vi "DutLug.vi"() -> (3 "histogram 2":T2(graph))   [LabVIEW 2019]
uses:
  <vilib>/Analysis/NI_AALBase.lvlib
panel:
  out "Cumulative count":cluster{"data sorted":dbl[], i32[]}(graph)
  out "sorted data":dbl[](graph)
  out "linear data out":dbl[](graph)
  out "Dynamic histogram out":T1(graph)
  out "histogram 1":T2(graph)
  in  "intervals":i32=200
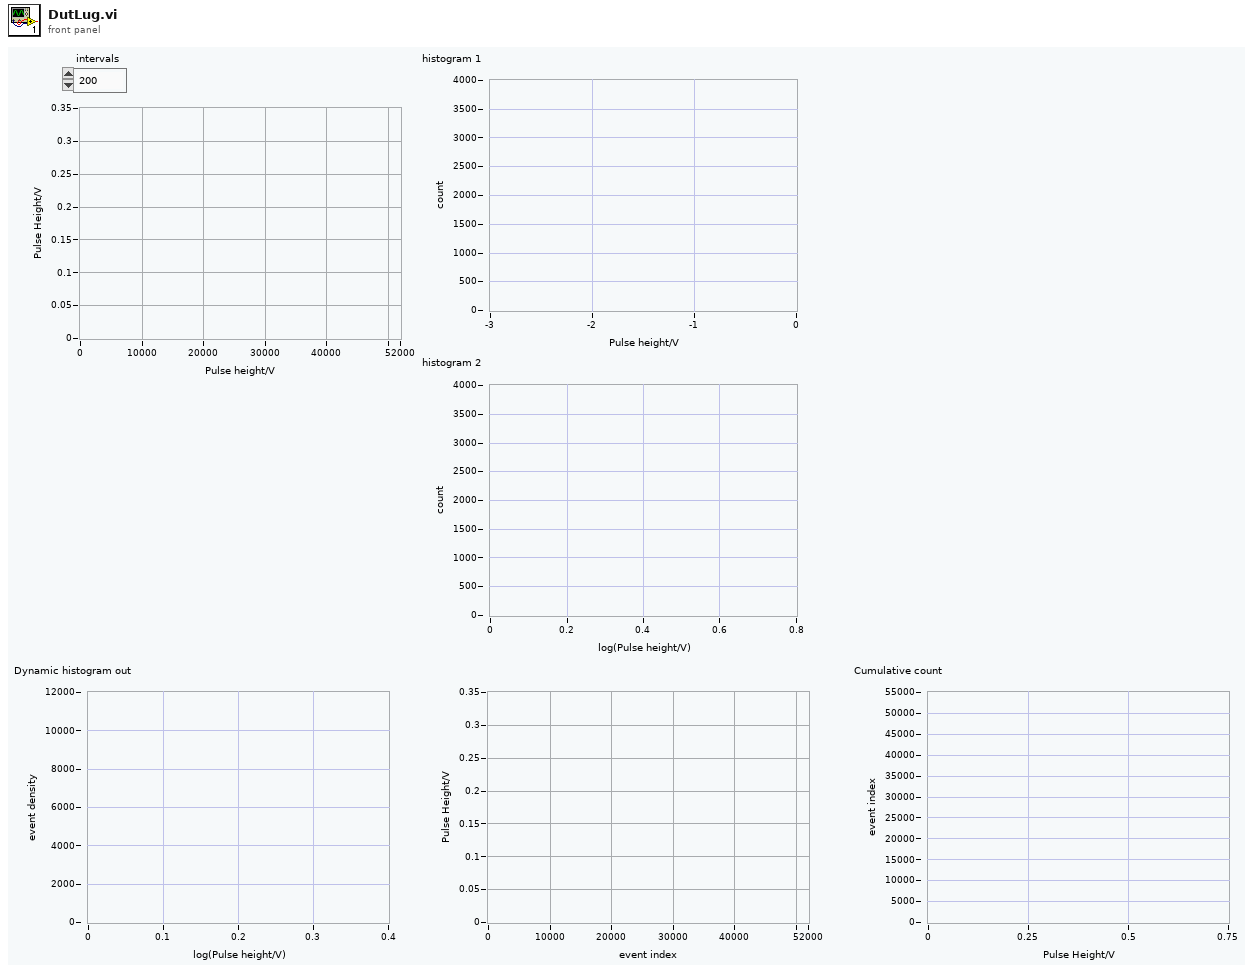
[diagram p1: front panel]
types:
  T1 = cluster{"Pulse amplitude":dbl[], "event density":dbl[]}
  T2 = cluster{"X Values":dbl[], "Histogram: h(x)":i32[]}
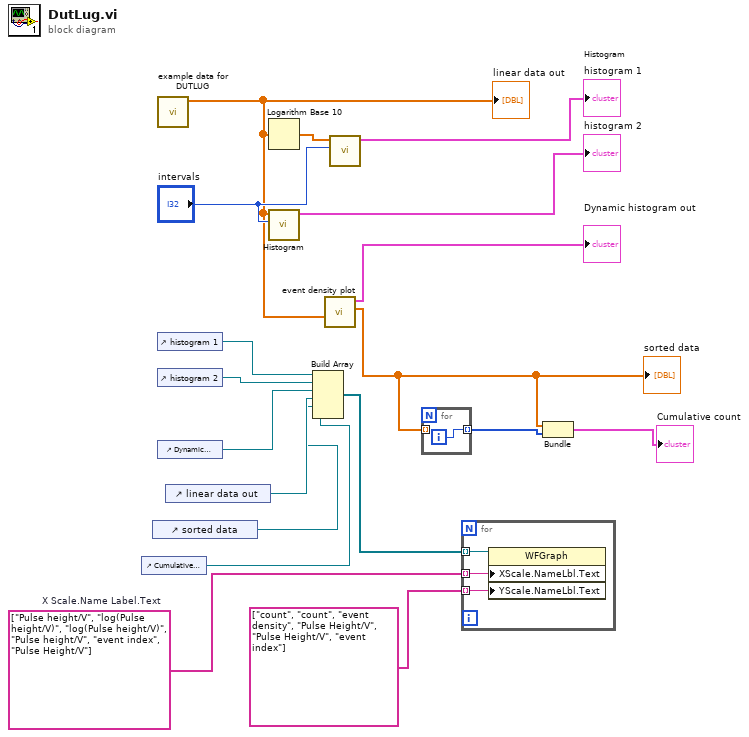
[diagram p0: block diagram]
diagram:
  w12 = string[] ["Pulse height/V", "log(Pulse height/V)", "log(Pulse height/V)", "Pulse height/V", "event index", "Pulse Height/V"]  # X Scale.Name Label.Text
  n1 = control-ref of="Cumulative count"() -> (w2:refnum<vi>)
  n2 = control-ref of="sorted data"() -> (w3:refnum<vi>)
  n3 = call "example data for DUTLUG.vi"() -> ("linear data out"=w14:dbl[])  [unwired: 11 in]
  "linear data out" <- w14
  n4 = control-ref of="histogram 1"() -> (w10:refnum<vi>)
  n5 = control-ref of="histogram 2"() -> (w9:refnum<vi>)
  n6 = control-ref of="Dynamic histogram out"() -> (w11:refnum<vi>)
  n7 = control-ref of="linear data out"() -> (w7:refnum<vi>)
  n8 = Logarithm Base 10(1:w14) -> (0:w16:dbl[])
  n9 = call <vilib>:"Histogram.vi"("intervals"="intervals", "X"=w14) -> ("Histogram Graph"=→"histogram 2":T2)  [unwired: 6 in, 3 out]
  n10 = Build Array(w10, w9, w11, w7, w3, w2) -> (w8:refnum<vi>[])
  n11 = call "event density plot.vi"("data in"=w14) -> ("data,sorted"=w5:dbl[], "Dynamic histogram out"=→"Dynamic histogram out":T1)  [unwired: 9 in]
  "sorted data" <- w5
  n12 = call <vilib>:"Histogram.vi"("intervals"="intervals", "X"=w16) -> ("Histogram Graph"=→"histogram 1":T2)  [unwired: 6 in, 3 out]
  n13 = for {
    tunnel: w5 -> [_] mode=indexing
    tunnel: [w19] -> w6 mode=indexing
    i -> [w19]
  }
  n14 = for {
    tunnel: w12 -> [w22] mode=indexing
    tunnel: w8 -> [w21] mode=indexing
    tunnel: string[] ["count", "count", "event density", "Pulse Height/V", "Pulse Height/V", "event index"] ("Array") -> [w20] mode=indexing
    n15 = property on="Property Node" class="WFGraph"(reference=w21, "XScale.NameLbl.Text"=w22, "YScale.NameLbl.Text"=w20) -> ()  [unwired: 1 in, 2 out]
  }
  n16 = Bundle("data,sorted"=w5, w6) -> (→"Cumulative count":cluster{"data,sorted":dbl[], i32[]})  [unwired: 1 in]
